vi "Test_WriteValue_InvalidRefnum_Error.vi"(8 "error in (no error)":errorcluster, 11 "TestCase in":refnum<class "TestTerminalVisibilityBinding.lvclass">) -> (0 "error out":errorcluster, 3 "TestCase out":refnum<class "TestTerminalVisibilityBinding.lvclass">)   [LabVIEW 2017, in "TestTerminalVisibilityBinding.lvclass"]
uses:
  TestTerminalVisibilityBinding.lvclass
  Source/Concrete/TerminalVisibilityBinding/TerminalVisibilityBinding.lvclass
  C:/Git/composed-transport/Source/ITransport/ITransport.lvclass
  Source/ITransport/ITransport.lvclass
panel:
  out "Return Error":errorcluster
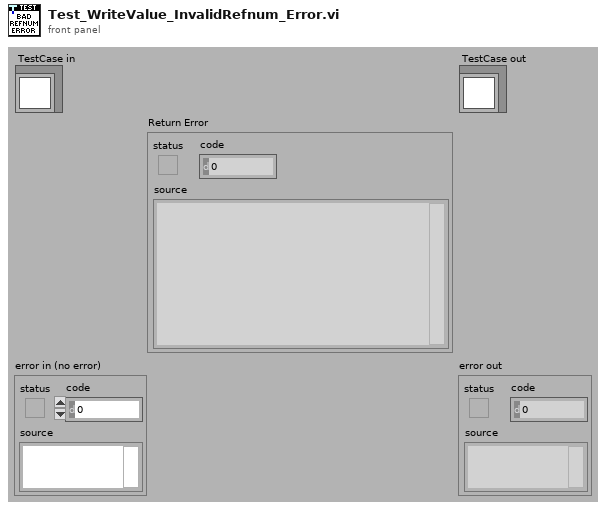
[diagram p1: front panel]
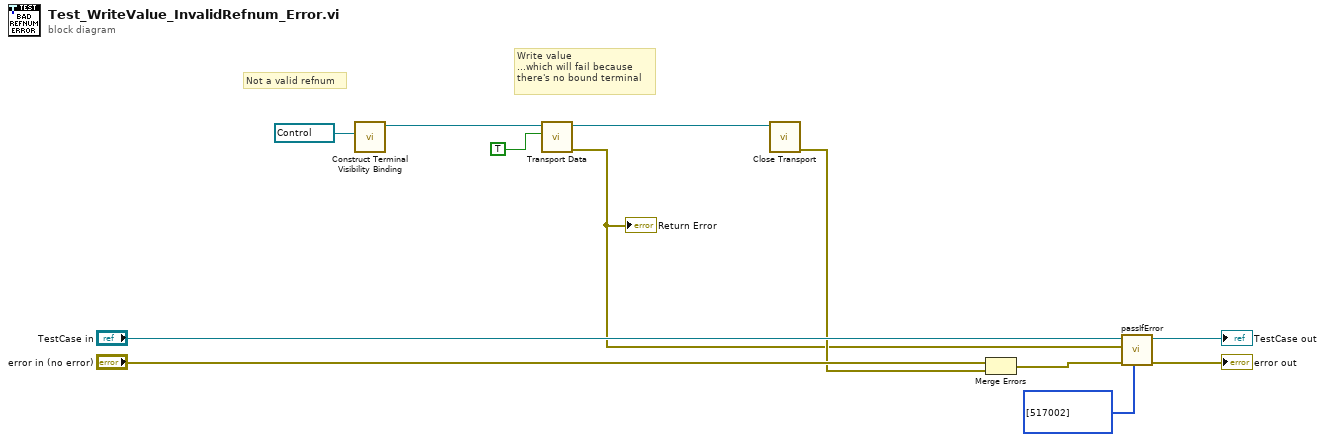
[diagram p0: block diagram]
diagram:
  # "Not a valid refnum"
  # "Write value\n...which will fail because\nthere's no bound terminal"
  n1 = call "Construct Terminal Visibility Binding.vi"("Ctl Refnum"=refnum<vi> refnum) -> ("TerminalVisibilityBinding"=w8:refnum<class "TerminalVisibilityBinding.lvclass">)  [unwired: 9 in, 1 out]
  n2 = call "Transport Data.vi"("Value"=TRUE, "ITransport in"=w8) -> ("error out"=w2:errorcluster, "ITransport out"=w5:refnum<class "TerminalVisibilityBinding.lvclass">)  [unwired: 8 in]
  "Return Error" <- w2
  n3 = call-dynamic "Close Transport.vi"("ITransport in"=w5) -> ("error out"=w4:errorcluster)  [unwired: 10 in]
  n4 = Merge Errors("error in (no error)", w4) -> (w7:errorcluster)
  n5 = call-dynamic "passIfError.vi"("passing error codes (default = any error code)"=i32[] [517002], "error in (no error)"=w7, "error"=w2, "TestCase in"="TestCase in") -> ("error out"=→"error out":errorcluster, "TestCase out"=→"TestCase out":refnum<class "TestTerminalVisibilityBinding.lvclass">)  [unwired: 6 in]
